vi "Sort Devices.vi"(8 "error in (no error)":errorcluster) -> (0 "error out":errorcluster, 3 "Devices (ordered)":tag[](array[tag]))   [LabVIEW 2019, in "Instrument.DAQ.lvclass"]
uses:
  Instrument.DAQ.lvclass
  <resource>/objmgr/daqmx.rc
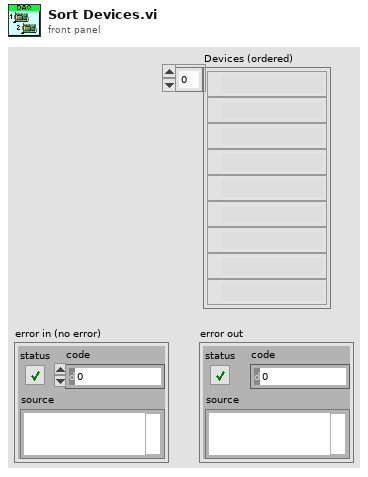
[diagram p1: front panel]
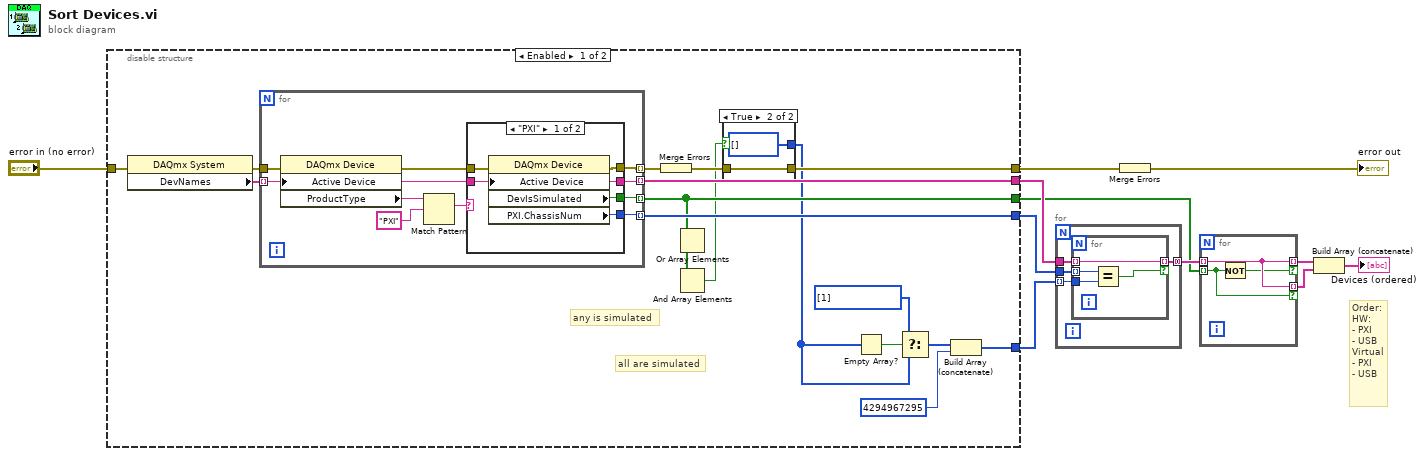
[diagram p0: block diagram]
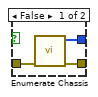
[diagram p2: hidden frame]
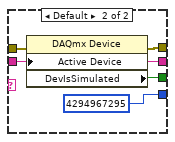
[diagram p3: hidden frame]
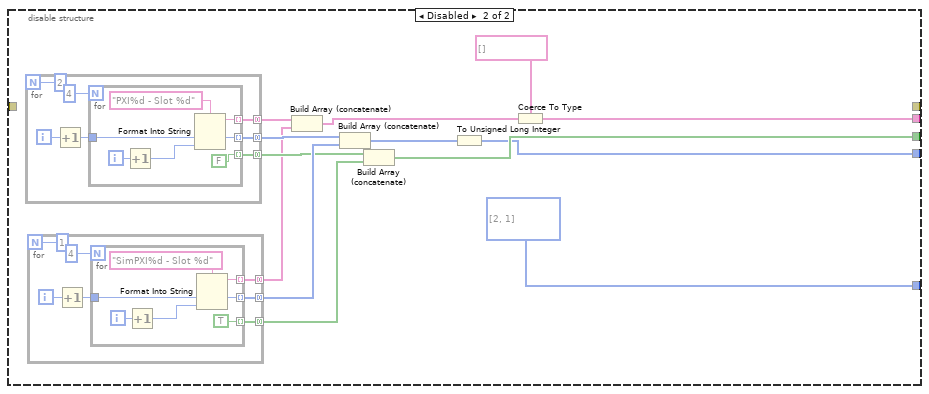
[diagram p4: hidden frame]
diagram:
  # "Order:\nHW:\n- PXI\n- USB\nVirtual\n- PXI\n- USB"
  n1 = disable-structure shown="Enabled" {
    disable-tunnel: "error in (no error)" -> [w15 _]
    disable-tunnel: [w16 _] -> w9
    disable-tunnel: [w22 u32[] [2, 1] ("PxiChassis Numbers")] -> w1
    disable-tunnel: [w27 w66] -> w7
    disable-tunnel: [w14 w54] -> w5
    disable-tunnel: [w24 w53] -> w8
    frame Enabled {
      # "all are simulated"
      # "any is simulated"
      n2 = property class="DAQmx System"(error in=w15) -> (error out=w26:errorcluster, "DevNames"=w25:tag[])  [unwired: 1 in, 1 out]
      n3 = for {
        tunnel: w25 -> [w34] mode=indexing
        tunnel: w26 -> [w42]
        tunnel: [w35] -> w18 mode=indexing
        tunnel: [w33] -> w27 mode=indexing
        tunnel: [w41] -> w14 mode=indexing
        tunnel: [w40] -> w24 mode=indexing
        n4 = property class="DAQmx Device"(error in=w42, "Active Device"=w34) -> (error out=w36:errorcluster, "ProductType"=w39:string)  [unwired: 1 in, 1 out]
        n5 = Match Pattern(string=w39, regular expression="PXI") -> (match substring=w38:string)  [unwired: 1 in, 3 out]
        n6 = case shown="\"PXI\"" w38 {
          tunnel: [w47 w52] -> w41
          tunnel: [w46 u32 4294967295 ("PXI.ChassisNum")] -> w40
          tunnel: w36 -> [w45 w50]
          tunnel: [w44 w51] -> w35
          tunnel: w34 -> [w43 w48]
          tunnel: [w43 w48] -> w33
          frame "PXI" {
            n7 = property class="DAQmx Device"(error in=w45, "Active Device"=w43) -> (error out=w44:errorcluster, "DevIsSimulated"=w47:bool, "PXI.ChassisNum"=w46:u32)  [unwired: 1 in, 1 out]
          }
          frame Default {
            n8 = property class="DAQmx Device"(error in=w50, "Active Device"=w48) -> (error out=w51:errorcluster, "DevIsSimulated"=w52:bool)  [unwired: 1 in, 1 out]
          }
        }
      }
      n9 = Merge Errors(w18) -> (w17:errorcluster)
      n10 = Or Array Elements(Boolean array=w14) -> ()  [unwired: 1 out]
      n11 = And Array Elements(Boolean array=w14) -> (logical AND=w12:bool)
      n12 = case shown="True" w12 {
        tunnel: w17 -> [w30 w32]
        tunnel: [w29 w32] -> w16
        tunnel: [w28 u32[] [] ("PxiChassisNumbers")] -> w13
        frame False {
          n13 = call "Enumerate Chassis.vi"("error in (no error)"=w30) -> ("error out"=w29:errorcluster, "PxiChassisNumbers"=w28:u32[])  [unwired: 9 in]
        }
        frame True {
        }
      }
      n14 = Empty Array?(array=w13) -> (empty?=w21:bool)
      n15 = Select(t=u32[] [1], s=w21, f=w13) -> (s? t:f=w19:u32[])
      n16 = Build Array (concatenate)(w19, u32 4294967295 ("x")) -> (w22:u32[])
    }
    frame Disabled {
      n17 = for {
        N: 2 -> [_]
        tunnel: [w85] -> w60 mode=concatenating
        tunnel: [w83] -> w59 mode=concatenating
        tunnel: [w80] -> w58 mode=concatenating
        i -> [w82]
        n18 = Increment(x=w82) -> (x+1=w81:i32)
        n19 = for {
          N: 4 -> [_]
          tunnel: [w90] -> w85 mode=indexing
          tunnel: w81 -> [w88]
          tunnel: [w88] -> w83 mode=indexing
          tunnel: [FALSE] -> w80 mode=indexing
          i -> [w91]
          n20 = Increment(x=w91) -> (x+1=w87:i32)
          n21 = Format Into String(format string="PXI%d - Slot %d", w88, w87) -> (resulting string=w90:string)  [unwired: 2 in, 1 out]
        }
      }
      n22 = for {
        N: 1 -> [_]
        tunnel: [w68] -> w57 mode=concatenating
        tunnel: [w72] -> w62 mode=concatenating
        tunnel: [w69] -> w61 mode=concatenating
        i -> [w71]
        n23 = Increment(x=w71) -> (x+1=w70:i32)
        n24 = for {
          N: 4 -> [_]
          tunnel: [w78] -> w68 mode=indexing
          tunnel: w70 -> [w76]
          tunnel: [w76] -> w72 mode=indexing
          tunnel: [TRUE] -> w69 mode=indexing
          i -> [w79]
          n25 = Increment(x=w79) -> (x+1=w75:i32)
          n26 = Format Into String(format string="SimPXI%d - Slot %d", w76, w75) -> (resulting string=w78:string)  [unwired: 2 in, 1 out]
        }
      }
      n27 = Build Array (concatenate)(w60, w57) -> (w55:string[])
      n28 = Build Array (concatenate)(w59, w62) -> (w56:i32[])
      n29 = Build Array (concatenate)(w58, w61) -> (w54:bool[])
      n30 = To Unsigned Long Integer(number=w56) -> (unsigned 32bit integer=w53:u32[])
      n31 = Coerce To Type(0:w55, 1:tag[] []) -> (2:w66:tag[])
    }
  }
  n32 = for {
    tunnel: w7 -> [w95]
    tunnel: w8 -> [w94]
    tunnel: [w93] -> w6 mode=concatenating
    tunnel: w1 -> [w92] mode=indexing
    n33 = for {
      tunnel: [w99] -> w93 mode=indexing if=w96
      tunnel: w95 -> [w99] mode=indexing
      tunnel: w94 -> [w98] mode=indexing
      tunnel: w92 -> [w97]
      n34 = Equal?(x=w98, y=w97) -> (x = y?=w96:bool)
    }
  }
  n35 = Merge Errors(w9) -> (→"error out":errorcluster)
  n36 = for {
    tunnel: [w102] -> w4 mode=indexing if=w101
    tunnel: w6 -> [w102] mode=indexing
    tunnel: [w102] -> w3 mode=indexing if=w100
    tunnel: w5 -> [w100] mode=indexing
    n37 = Not(x=w100) -> (.not. x?=w101:bool)
  }
  n38 = Build Array (concatenate)(w4, w3) -> (→"Devices (ordered)":tag[])
